vi "Read Serial Number.vi"() -> (3 "serial number":string)   [LabVIEW 2020]
uses:
  <vilib>/Utility/config.llb/Read Key (String).vi
  <vilib>/Utility/config.llb/NI_LVConfig.lvlib
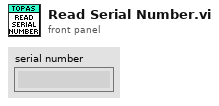
[diagram p1: front panel]
types:
  T1 = typedef "NI_LVConfig.lvlib/Config Data RefNum.ctl" = refnum<k1>
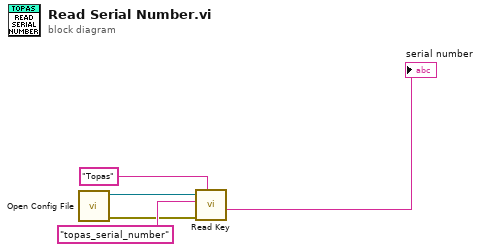
[diagram p0: block diagram]
diagram:
  n1 = call "Open Config File.vi"() -> ("error out"=w2:errorcluster, "Refnum out"=w1:T1)  [unwired: 10 in]
  n2 = call-poly <vilib>:"Read Key.vi"("section"="Topas", "error in (no error)"=w2, "key"="topas_serial_number", "refnum"=w1) -> ("value"=→"serial number":string)  [unwired: 4 in, 3 out]
